vi "Write script.vi"(8 "error in (no error)":errorcluster caption="에러 입력(에러 없음)", 10 "script":string, 11 "Script Line 입력":refnum<class "Script Line.lvclass">) -> (0 "error out":errorcluster caption="에러 출력", 3 "Script Line 출력":refnum<class "Script Line.lvclass">)   [LabVIEW 2020, in "Script Line.lvclass"]
uses:
  Script Line.lvclass
  Script Line.lvclass/Script Line.ctl
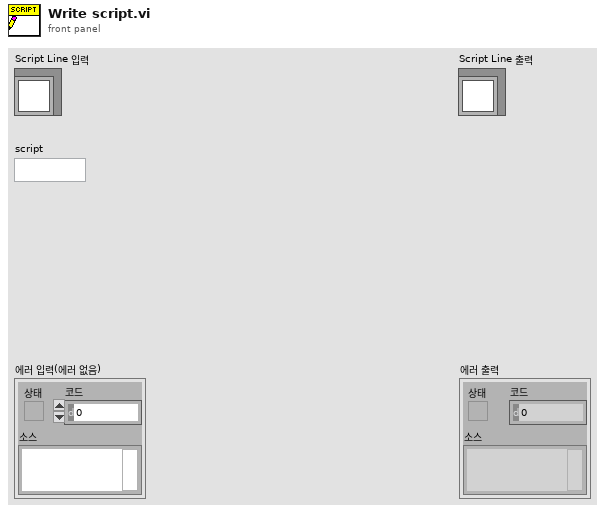
[diagram p1: front panel]
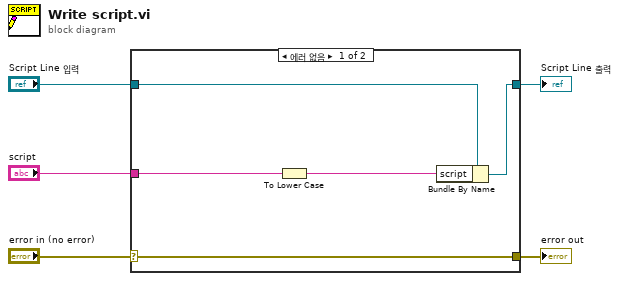
[diagram p0: block diagram]
diagram:
  n1 = case shown="에러 없음" "error in (no error)" {
    selector: "error in (no error)" -> [w10 w11]
    tunnel: [w10 w11] -> w4
    tunnel: [w8 w12] -> w2
    tunnel: "Script Line 입력" -> [w9 w12]
    tunnel: "script" -> [w7 _]
    frame No Error {
      n2 = To Lower Case(string=w7) -> (all lower case string=w6:string)
      n3 = Bundle By Name(cluster=w9, "script"=w6) -> (w8:refnum<class "Script Line.lvclass">)
    }
    frame Error {
    }
  }
  "error out" <- w4
  "Script Line 출력" <- w2
